vi "GenerateDisplay 1-1.vi"() -> ()   [LabVIEW 2018]
doc: "该模板可用于模拟数据的生成与显示。\n注: 通过该模板创建的VI中，默认情况下LabVIEW将启用自动错误处理。"
uses:
  Instance           1 27Saved   GenerateDisplay.vit .vi
panel:
  out "Waveform Graph":dynamicdata(graph) caption="波形图"
  in  "stop":bool caption="停止"
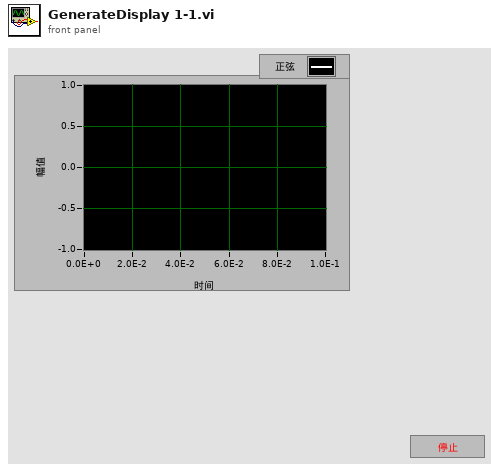
[diagram p1: front panel]
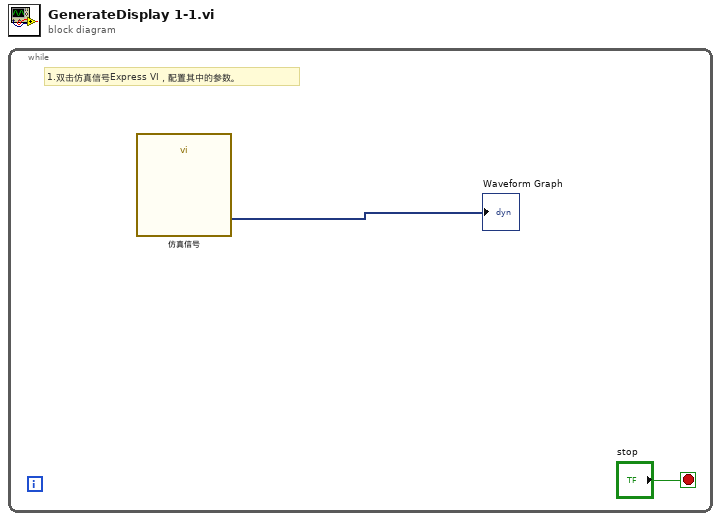
[diagram p0: block diagram]
diagram:
  n1 = while {
    stop <- "stop" stop-if-true
    # "1.双击仿真信号Express VI，配置其中的参数。"
    n2 = call "仿真信号"() -> ("Sine"=→"Waveform Graph":dynamicdata)  [unwired: 14 in, 1 out]
  }
